vi "Number of IMages in Current Set.vi"(8 "Error In":errorcluster) -> (0 "Error Out":errorcluster, 3 "Number of pics taken Out":i32)   [LabVIEW 2014]
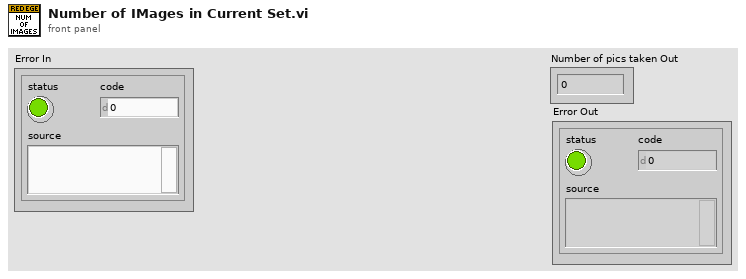
[diagram p1: front panel]
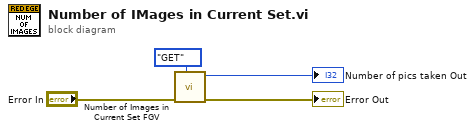
[diagram p0: block diagram]
diagram:
  n1 = call "Number of Images in Current Set FGV.vi"("Operation"=enum16{"GET", "SET"}."GET", "Error In"="Error In") -> ("Error Out"=→"Error Out":errorcluster, "Number of pics taken Out"=→"Number of pics taken Out":i32)  [unwired: 8 in]
